vi "Read Serial Device.lvclass.vi"(8 "error in (no error)":errorcluster, 11 "UI Actor in":refnum<class "UI Actor.lvclass">) -> (0 "error out":errorcluster, 2 "Serial Device.lvclass":refnum<class "Serial Device.lvclass">, 3 "UI Actor out":refnum<class "UI Actor.lvclass">)   [LabVIEW 2020, in "UI Actor.lvlib" / "UI Actor.lvclass"]
uses:
  UI Actor.lvclass
  Abstract/Serial Device/Serial Device.lvclass
  UI Actor.lvclass/UI Actor.ctl
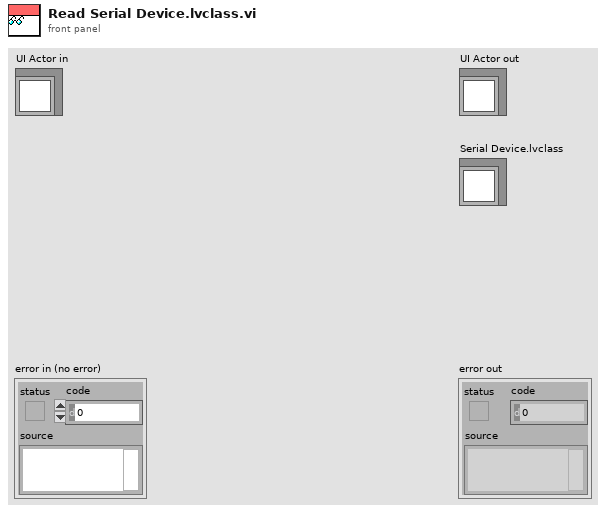
[diagram p1: front panel]
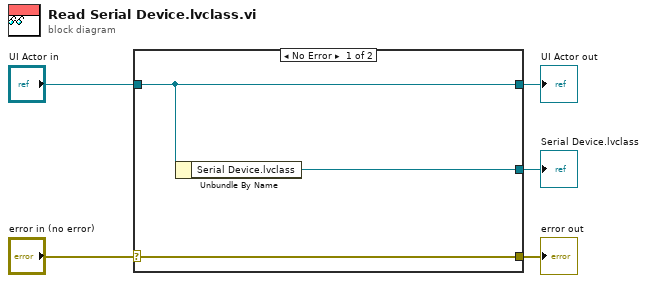
[diagram p0: block diagram]
diagram:
  n1 = case shown="No Error" "error in (no error)" {
    selector: "error in (no error)" -> [w8 w9]
    tunnel: [w8 w9] -> w4
    tunnel: [w7 w10] -> w2
    tunnel: "UI Actor in" -> [w7 w10]
    tunnel: [w6 _] -> w1
    frame No Error {
      n2 = Unbundle By Name(w7) -> ("Serial Device.lvclass"=w6:refnum<class "Serial Device.lvclass">)
    }
    frame Error {
    }
  }
  "error out" <- w4
  "UI Actor out" <- w2
  "Serial Device.lvclass" <- w1
